vi "sub_create save files.vi"(5 "# of Quick Restarts":i32) -> (0 "error out":errorcluster, 1 "Peltier Save Files":path[](array[path]), 2 "Save Path":path)   [LabVIEW 2021]
uses:
  globalvariables.vi
  <vilib>/Utility/file.llb/Write Delimited Spreadsheet (string).vi
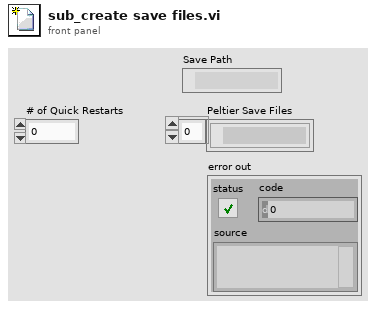
[diagram p1: front panel]
types:
  T1 = enum16{"open", "replace", "create", "open or create", "replace or create", "replace or create with confirmation"}
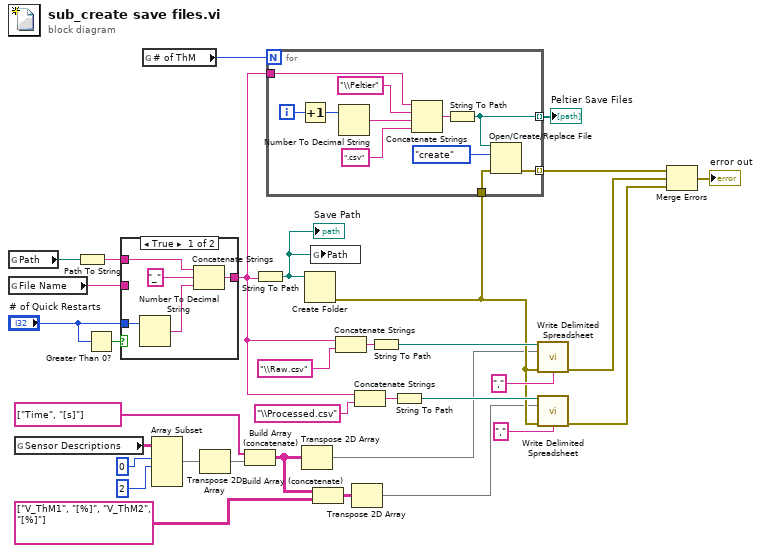
[diagram p0: block diagram]
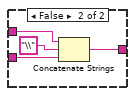
[diagram p2: hidden frame]
diagram:
  n1 = global read "globalvariables.vi" "Path"() -> (w23:path)
  n2 = global read "globalvariables.vi" "File Name"() -> (w27:string)
  n3 = global read "globalvariables.vi" "Sensor Descriptions"() -> (w11:string[][])
  n4 = Path To String(path=w23) -> (string=w22:string)
  n5 = Greater Than 0?(x="# of Quick Restarts") -> (x > 0?=w1:bool)
  n6 = case shown="True" w1 {
    tunnel: w27 -> [_ w42]
    tunnel: [w34 w41] -> w20
    tunnel: "# of Quick Restarts" -> [w38 _]
    tunnel: w22 -> [w35 w39]
    frame True {
      n7 = Number To Decimal String(number=w38) -> (decimal integer string=w36:string)  [unwired: 1 in]
      n8 = Concatenate Strings(w35, "_", w36) -> (w34:string)
    }
    frame False {
      n9 = Concatenate Strings(w39, "\\", w42) -> (w41:string)
    }
  }
  n10 = global read "globalvariables.vi" "# of ThM"() -> (w24:i32)
  n11 = Array Subset(array=w11, index (row)=0, length (row)=2) -> (w9:string[][])  [unwired: 2 in]
  n12 = Transpose 2D Array(2D array=w9) -> (transposed array=w8:string[][])
  n13 = Build Array (concatenate)(string[] ["Time", "[s]"], w8) -> (w7:string[][])
  n14 = String To Path(string=w20) -> (path=w21:path)
  "Save Path" <- w21
  n15 = Transpose 2D Array(2D array=w7) -> (transposed array=w4:string[][])
  n16 = Create Folder(path (use dialog)=w21) -> (error out=w14:errorcluster)  [unwired: 2 in, 2 out]
  n17 = for {
    N: w24 -> [_]
    tunnel: w20 -> [w50]
    tunnel: [w47] -> w19 mode=indexing
    tunnel: [w44] -> w18 mode=indexing
    tunnel: w14 -> [w43]
    i -> [w45]
    n18 = Increment(x=w45) -> (x+1=w46:i32)
    n19 = Number To Decimal String(number=w46) -> (decimal integer string=w52:string)  [unwired: 1 in]
    n20 = Concatenate Strings(w50, "\\Peltier", w52, ".csv") -> (w48:string)
    n21 = String To Path(string=w48) -> (path=w47:path)
    n22 = Open/Create/Replace File(file path (use dialog)=w47, error in=w43, operation (0:open)=T1."create") -> (error out=w44:errorcluster)  [unwired: 3 in, 2 out]
  }
  "Peltier Save Files" <- w19
  n23 = global write "globalvariables.vi" "Path"(w21) -> ()
  n24 = Build Array (concatenate)(w7, string[][] [["V_ThM1", "[%]"], ["V_ThM2", "[%]"]]) -> (w5:string[][])
  n25 = Concatenate Strings(w20, "\\Raw.csv") -> (w30:string)
  n26 = Transpose 2D Array(2D array=w5) -> (transposed array=w3:string[][])
  n27 = Concatenate Strings(w20, "\\Processed.csv") -> (w31:string)
  n28 = String To Path(string=w30) -> (path=w28:path)
  n29 = String To Path(string=w31) -> (path=w29:path)
  n30 = call-poly <vilib>:"Write Delimited Spreadsheet.vi"("file path (dialog if empty)"=w28, "2D data"=w4, "error in (no error)"=w14, "delimiter (\\t)"=",") -> ("error out"=w17:errorcluster)  [unwired: 10 in, 1 out]
  n31 = call-poly <vilib>:"Write Delimited Spreadsheet.vi"("file path (dialog if empty)"=w29, "2D data"=w3, "error in (no error)"=w14, "delimiter (\\t)"=",") -> ("error out"=w16:errorcluster)  [unwired: 10 in, 1 out]
  n32 = Merge Errors(w18, w17, w16) -> (→"error out":errorcluster)
